vi "runtime test.vi"() -> (0 "error out":errorcluster, 2 "success?":bool)   [LabVIEW 2014, in "Shared Memory tests.lvlib"]
uses:
  Shared Memory tests.lvlib
  module/execution/Shared Memory runtime.lvclass
  <vilib>/NI/Tag Bus Module Framework/channel/channel classification.ctl
  module/execution/Shared Memory runtime.lvclass/Shared Memory runtime.ctl
  <vilib>/NI/NI Linux RT IPC/Shared Memory/Pointer Operations/Read 1D Array DBL.vi
  <vilib>/NI/Tag Bus/table/write multiple elements.vi
  <vilib>/NI/Tag Bus/table/data polymorphs/write many/write Doubles.vi
  <vilib>/NI/NI Linux RT IPC/Shared Memory/Pointer Operations/Read 1D Array SGL.vi
  <vilib>/NI/Tag Bus/table/data polymorphs/write many/write Singles.vi
  <vilib>/NI/NI Linux RT IPC/Shared Memory/Pointer Operations/Read 1D Array I64.vi
  <vilib>/NI/Tag Bus/table/data polymorphs/write many/write I64s.vi
  <vilib>/NI/NI Linux RT IPC/Shared Memory/Pointer Operations/Read 1D Array I32.vi
  <vilib>/NI/Tag Bus/table/data polymorphs/write many/write I32s.vi
  <vilib>/NI/NI Linux RT IPC/Shared Memory/Pointer Operations/Read 1D Array I16.vi
  <vilib>/NI/Tag Bus/table/data polymorphs/write many/write I16s.vi
  <vilib>/NI/NI Linux RT IPC/Shared Memory/Pointer Operations/Read 1D Array I8.vi
  <vilib>/NI/Tag Bus/table/data polymorphs/write many/write I8s.vi
  <vilib>/NI/NI Linux RT IPC/Shared Memory/Pointer Operations/Read 1D Array U64.vi
  <vilib>/NI/Tag Bus/table/data polymorphs/write many/write U64s.vi
  <vilib>/NI/NI Linux RT IPC/Shared Memory/Pointer Operations/Read 1D Array U32.vi
  <vilib>/NI/Tag Bus/table/data polymorphs/write many/write U32s.vi
  <vilib>/NI/NI Linux RT IPC/Shared Memory/Pointer Operations/Read 1D Array U16.vi
  <vilib>/NI/Tag Bus/table/data polymorphs/write many/write U16s.vi
  <vilib>/NI/NI Linux RT IPC/Shared Memory/Pointer Operations/Read 1D Array U8.vi
  <vilib>/NI/Tag Bus/table/data polymorphs/write many/write U8s.vi
  <vilib>/NI/NI Linux RT IPC/Shared Memory/Pointer Operations/Read 1D Array Boolean.vi
  <vilib>/NI/Tag Bus/table/data polymorphs/write many/write Booleans.vi
  <vilib>/NI/Tag Bus/table/write sequential data elements.vi
  <vilib>/NI/Tag Bus/table/data polymorphs/write sequential/write sequential Doubles.vi
  <vilib>/NI/Tag Bus/table/data polymorphs/write sequential/write sequential Singles.vi
  <vilib>/NI/Tag Bus/table/data polymorphs/write sequential/write sequential I64s.vi
  <vilib>/NI/Tag Bus/table/data polymorphs/write sequential/write sequential I32s.vi
  <vilib>/NI/Tag Bus/table/data polymorphs/write sequential/write sequential I16s.vi
  <vilib>/NI/Tag Bus/table/data polymorphs/write sequential/write sequential I8s.vi
  <vilib>/NI/Tag Bus/table/data polymorphs/write sequential/write sequential U64s.vi
  <vilib>/NI/Tag Bus/table/data polymorphs/write sequential/write sequential U32s.vi
  <vilib>/NI/Tag Bus/table/data polymorphs/write sequential/write sequential U16s.vi
  <vilib>/NI/Tag Bus/table/data polymorphs/write sequential/write sequential U8s.vi
  <vilib>/NI/Tag Bus/table/data polymorphs/write sequential/write sequential Booleans.vi
  module/execution/read channels of classification.vi
  <vilib>/NI/Tag Bus/table/read multiple elements.vi
  <vilib>/NI/Tag Bus/table/data polymorphs/read many/read Doubles.vi
  <vilib>/NI/NI Linux RT IPC/Shared Memory/Pointer Operations/Write 1D Array DBL.vi
  <vilib>/NI/Tag Bus/table/data polymorphs/read many/read Singles.vi
  <vilib>/NI/NI Linux RT IPC/Shared Memory/Pointer Operations/Write 1D Array SGL.vi
  <vilib>/NI/Tag Bus/table/data polymorphs/read many/read I64s.vi
  <vilib>/NI/NI Linux RT IPC/Shared Memory/Pointer Operations/Write 1D Array I64.vi
  <vilib>/NI/Tag Bus/table/data polymorphs/read many/read I32s.vi
  <vilib>/NI/NI Linux RT IPC/Shared Memory/Pointer Operations/Write 1D Array I32.vi
  <vilib>/NI/Tag Bus/table/data polymorphs/read many/read I16s.vi
  <vilib>/NI/NI Linux RT IPC/Shared Memory/Pointer Operations/Write 1D Array I16.vi
  <vilib>/NI/Tag Bus/table/data polymorphs/read many/read I8s.vi
  <vilib>/NI/NI Linux RT IPC/Shared Memory/Pointer Operations/Write 1D Array I8.vi
  <vilib>/NI/Tag Bus/table/data polymorphs/read many/read U64s.vi
  <vilib>/NI/NI Linux RT IPC/Shared Memory/Pointer Operations/Write 1D Array U64.vi
  <vilib>/NI/Tag Bus/table/data polymorphs/read many/read U32s.vi
  <vilib>/NI/NI Linux RT IPC/Shared Memory/Pointer Operations/Write 1D Array U32.vi
  <vilib>/NI/Tag Bus/table/data polymorphs/read many/read U16s.vi
  <vilib>/NI/NI Linux RT IPC/Shared Memory/Pointer Operations/Write 1D Array U16.vi
  <vilib>/NI/Tag Bus/table/data polymorphs/read many/read U8s.vi
  <vilib>/NI/NI Linux RT IPC/Shared Memory/Pointer Operations/Write 1D Array U8.vi
  <vilib>/NI/Tag Bus/table/data polymorphs/read many/read Booleans.vi
  <vilib>/NI/NI Linux RT IPC/Shared Memory/Pointer Operations/Write 1D Array Boolean.vi
  <vilib>/NI/Tag Bus/table/read sequential data elements.vi
  <vilib>/NI/Tag Bus/table/data polymorphs/read sequential/read sequential Doubles.vi
  <vilib>/NI/Tag Bus/table/data polymorphs/read sequential/read sequential Singles.vi
  <vilib>/NI/Tag Bus/table/data polymorphs/read sequential/read sequential I64s.vi
  <vilib>/NI/Tag Bus/table/data polymorphs/read sequential/read sequential I32s.vi
  <vilib>/NI/Tag Bus/table/data polymorphs/read sequential/read sequential I16s.vi
  <vilib>/NI/Tag Bus/table/data polymorphs/read sequential/read sequential I8s.vi
  <vilib>/NI/Tag Bus/table/data polymorphs/read sequential/read sequential U64s.vi
  <vilib>/NI/Tag Bus/table/data polymorphs/read sequential/read sequential U32s.vi
  <vilib>/NI/Tag Bus/table/data polymorphs/read sequential/read sequential U16s.vi
  <vilib>/NI/Tag Bus/table/data polymorphs/read sequential/read sequential U8s.vi
  <vilib>/NI/Tag Bus/table/data polymorphs/read sequential/read sequential Booleans.vi
  module/execution/Read input data.vi
  module/execution/Read processing parameters.vi
  module/execution/Read processing results.vi
  module/execution/Read output data.vi
  <vilib>/NI/NI Linux RT IPC/Shared Memory/Classes/Shared Memory/Shared Memory.lvclass
  module/configuration/Shared Memory configuration.lvclass
  <vilib>/NI/Tag Bus Module Framework/channel/TBM channel.lvclass
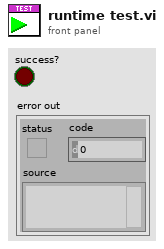
[diagram p1: front panel]
types:
  T1 = typedef "TBM channel.lvclass/channel classification.ctl" = enum16{"input data", "output data", "processing parameter", "processing result"}
  T2 = typedef "TBM channel.lvclass/data tables.ctl" = cluster{"input data":T3, "processing parameter":T3, "processing result":T3, "output data":T3}
  T3 = typedef "tag bus.lvlib/dictionary table pair.ctl" = cluster{"data dictionary":refnum<class "data dictionary.lvclass">, "data table":T4}
  T4 = typedef "tag bus.lvlib/data table.lvlib/data table.ctl" = cluster{"Double":dbl[], "Single":sgl[], "I64":i64[], "I32":i32[], "I16":i16[], "I8":i8[], "U64":u64[], "U32":u32[], "U16":u16[], "U8":u8[], "Boolean":bool[], "String":string[], "Array of Double":cluster{"DBL Array":dbl[]}[], "Array of Single":cluster{"SGL Array":sgl[]}[], "Array of I64":cluster{"I64 Array":i64[]}[], "Array of I32":cluster{"I32 Array":i32[]}[], "Array of I16":cluster{"I16 Array":i16[]}[], "Array of I8":cluster{"I8 Array":i8[]}[], "Array of U64":cluster{"U64 Array":u64[]}[], "Array of U32":cluster{"U32 Array":u32[]}[], "Array of U16":cluster{"U16 Array":u16[]}[], "Array of U8":cluster{"U8 Array":u8[]}[], "Array of Boolean":cluster{"Boolean Array":bool[]}[], "Array of String":cluster{"String Array":string[]}[]}
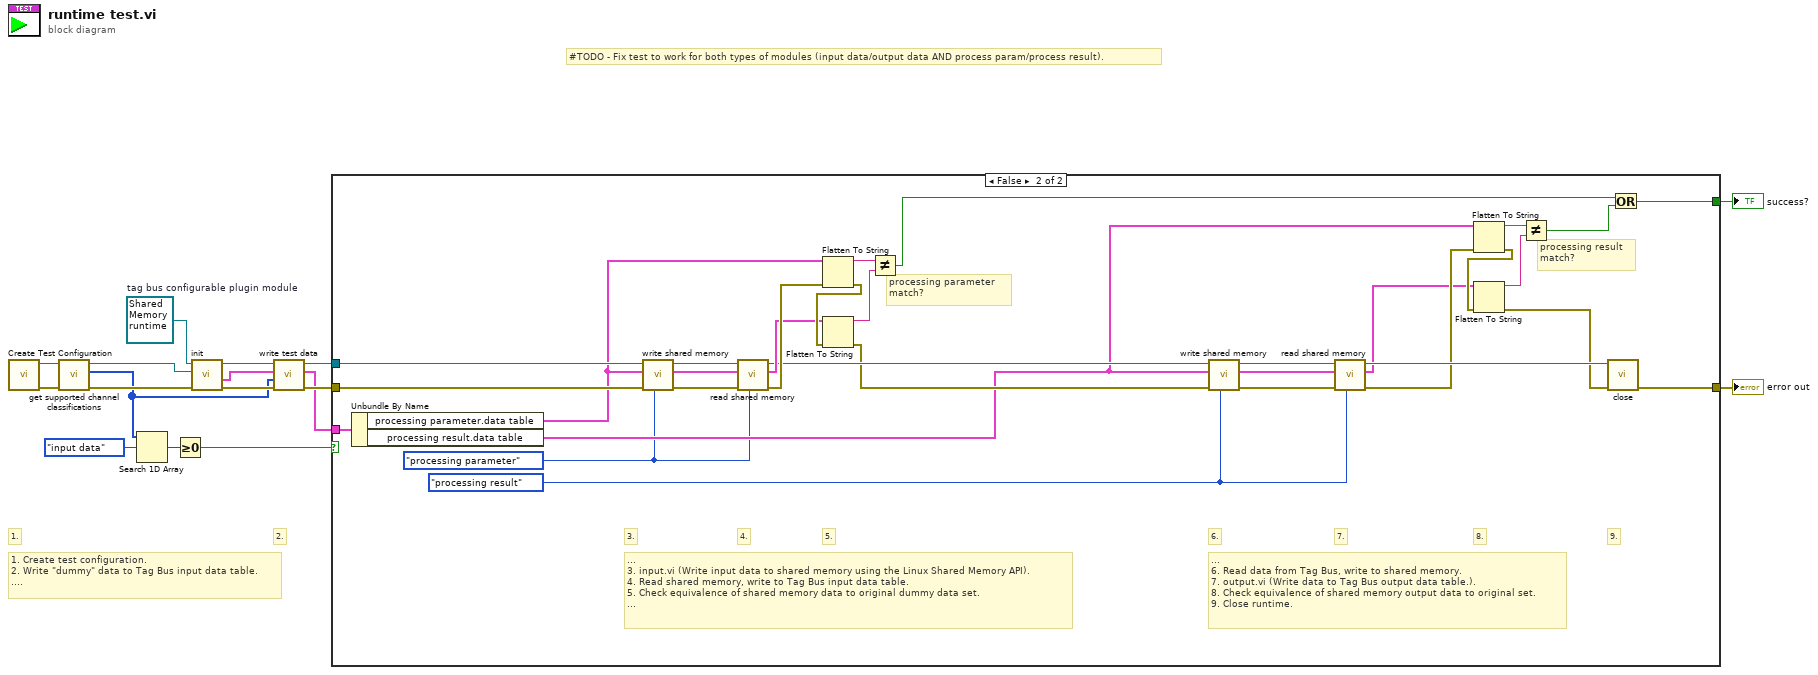
[diagram p0: block diagram]
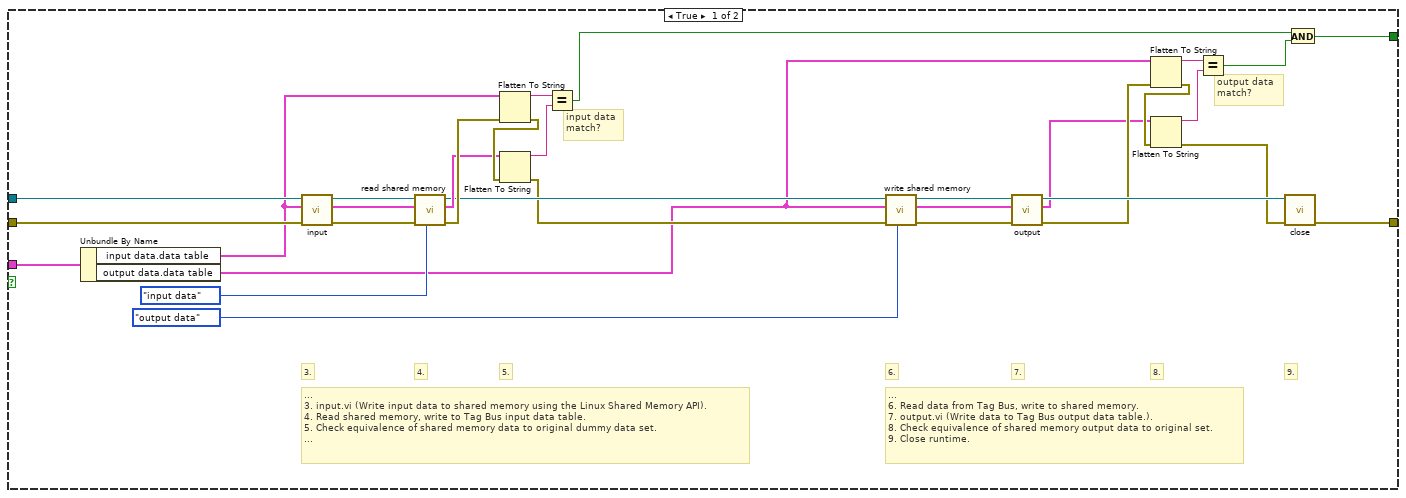
[diagram p2: hidden frame]
diagram:
  w13 = refnum<class "Shared Memory runtime.lvclass"> refnum  # tag bus configurable plugin module
  # "#TODO - Fix test to work for both types of modules (input data/output data AND process param/process result)."
  # "2."
  # "1. Create test configuration.\n2. Write \"dummy\" data to Tag Bus input data table.\n...."
  # "1."
  n1 = call "Create Test Configuration.vi"() -> ("error out"=w15:errorcluster, "Module Configuration"=w14:refnum<class "Shared Memory configuration.lvclass">)  [unwired: 3 in, 7 out]
  n2 = call-dynamic "get supported channel classifications.vi"("error in"=w15, "module configuration in"=w14) -> ("error out"=w12:errorcluster, "supported classes"=w5:T1[], "module configuration out"=w11:refnum<class "Shared Memory configuration.lvclass">)  [unwired: 7 in]
  n3 = Search 1D Array(1D array=w5, element=channel_classification."input data" ("channel classification")) -> (index of element=w3:i32)  [unwired: 1 in]
  n4 = Greater Or Equal To 0?(x=w3) -> (x >= 0?=w1:bool)
  n5 = call-dynamic "init.vi"("error in"=w12, "TBM module configuration in"=w11, "Shared Memory runtime in"=w13) -> ("error out"=w8:errorcluster, "data allocations"=w6:T2, "Shared Memory runtime out"=w7:refnum<class "Shared Memory runtime.lvclass">)  [unwired: 5 in, 1 out]
  n6 = call "write test data.vi"("shared memory runtime"=w7, "data allocations"=w6, "supported classifications"=w5, "error in"=w8) -> ("shared memory runtime out"=w9:refnum<class "Shared Memory runtime.lvclass">, "data allocations out"=w2:T2, "error out"=w10:errorcluster)  [unwired: 4 in]
  n7 = case shown="False" w1 {
    tunnel: [w48 w79] -> w17
    tunnel: [w47 w78] -> w16
    tunnel: w10 -> [w42 w54]
    tunnel: w9 -> [w41 w56]
    tunnel: w2 -> [w19 w58]
    frame True {
      # "output data\nmatch?"
      # "input data\nmatch?"
      # "...\n6. Read data from Tag Bus, write to shared memory.\n7. output.vi (Write data to Tag Bus output data table.).\n8. Check equivalence of shared memory output data to original set.\n9. Close runtime."
      # "...\n3. input.vi (Write input data to shared memory using the Linux Shared Memory API).\n4. Read shared memory, write to Tag Bus input data table.\n5. Check equivalence of shared memory data to original dummy data set.\n..."
      # "6."
      # "5."
      # "7."
      # "4."
      # "3."
      # "8."
      # "9."
      n8 = Unbundle By Name(w19) -> ("input data.data table"=w20:T4, "output data.data table"=w18:T4)
      n9 = call-dynamic "input.vi"("error in"=w42, "data table in"=w20, "Shared Memory runtime in"=w41) -> ("error out"=w37:errorcluster, "data table out"=w31:T4, "Shared Memory runtime out"=w36:refnum<class "Shared Memory runtime.lvclass">)  [unwired: 6 in]
      n10 = call "read shared memory.vi"("channel classification"=channel_classification."input data", "error in"=w37, "data table"=w31, "Shared Memory runtime"=w36) -> ("error out"=w35:errorcluster, "data table out"=w34:T4, "Shared Memory runtime out"=w33:refnum<class "Shared Memory runtime.lvclass">)  [unwired: 5 in]
      n11 = Flatten To String(anything=w20, error in (no error)=w35) -> (data string=w40:string, error out=w38:errorcluster)  [unwired: 2 in, 1 out]
      n12 = Flatten To String(anything=w34, error in (no error)=w38) -> (data string=w39:string, error out=w32:errorcluster)  [unwired: 2 in, 1 out]
      n13 = Equal?(x=w40, y=w39) -> (x = y?=w45:bool)
      n14 = call "write shared memory.vi"("channel classification"=channel_classification."output data", "error in"=w32, "data table"=w18, "module in"=w33) -> ("error out"=w29:errorcluster, "data table out"=w23:T4, "module out"=w30:refnum<class "Shared Memory runtime.lvclass">)  [unwired: 5 in]
      n15 = call-dynamic "output.vi"("error in"=w29, "data table in"=w23, "Shared Memory runtime in"=w30) -> ("error out"=w25:errorcluster, "data table out"=w24:T4, "Shared Memory runtime out"=w46:refnum<class "Shared Memory runtime.lvclass">)  [unwired: 6 in]
      n16 = Flatten To String(anything=w18, error in (no error)=w25) -> (data string=w26:string, error out=w28:errorcluster)  [unwired: 2 in, 1 out]
      n17 = Flatten To String(anything=w24, error in (no error)=w28) -> (data string=w27:string, error out=w43:errorcluster)  [unwired: 2 in, 1 out]
      n18 = Equal?(x=w26, y=w27) -> (x = y?=w44:bool)
      n19 = call-dynamic "close.vi"("error in"=w43, "Shared Memory runtime in"=w46) -> ("error out"=w48:errorcluster)  [unwired: 9 in]
      n20 = And(x=w45, y=w44) -> (x .and. y?=w47:bool)
    }
    frame False {
      w50 = channel_classification."processing result" ("channel classification")
      w52 = channel_classification."processing parameter" ("channel classification")
      # "processing result\nmatch?"
      # "processing parameter\nmatch?"
      # "...\n6. Read data from Tag Bus, write to shared memory.\n7. output.vi (Write data to Tag Bus output data table.).\n8. Check equivalence of shared memory output data to original set.\n9. Close runtime."
      # "...\n3. input.vi (Write input data to shared memory using the Linux Shared Memory API).\n4. Read shared memory, write to Tag Bus input data table.\n5. Check equivalence of shared memory data to original dummy data set.\n..."
      # "6."
      # "5."
      # "7."
      # "4."
      # "3."
      # "8."
      # "9."
      n21 = Unbundle By Name(w58) -> ("processing parameter.data table"=w49:T4, "processing result.data table"=w57:T4)
      n22 = call "write shared memory.vi"("channel classification"=w52, "error in"=w54, "data table"=w49, "module in"=w56) -> ("error out"=w53:errorcluster, "data table out"=w51:T4, "module out"=w55:refnum<class "Shared Memory runtime.lvclass">)  [unwired: 5 in]
      n23 = call "read shared memory.vi"("channel classification"=w52, "error in"=w53, "data table"=w51, "Shared Memory runtime"=w55) -> ("error out"=w70:errorcluster, "data table out"=w69:T4, "Shared Memory runtime out"=w68:refnum<class "Shared Memory runtime.lvclass">)  [unwired: 5 in]
      n24 = Flatten To String(anything=w49, error in (no error)=w70) -> (data string=w73:string, error out=w71:errorcluster)  [unwired: 2 in, 1 out]
      n25 = Flatten To String(anything=w69, error in (no error)=w71) -> (data string=w72:string, error out=w67:errorcluster)  [unwired: 2 in, 1 out]
      n26 = Not Equal?(x=w73, y=w72) -> (x != y?=w76:bool)
      n27 = call "write shared memory.vi"("channel classification"=w50, "error in"=w67, "data table"=w57, "module in"=w68) -> ("error out"=w65:errorcluster, "data table out"=w59:T4, "module out"=w66:refnum<class "Shared Memory runtime.lvclass">)  [unwired: 5 in]
      n28 = call "read shared memory.vi"("channel classification"=w50, "error in"=w65, "data table"=w59, "Shared Memory runtime"=w66) -> ("error out"=w61:errorcluster, "data table out"=w60:T4, "Shared Memory runtime out"=w77:refnum<class "Shared Memory runtime.lvclass">)  [unwired: 5 in]
      n29 = Flatten To String(anything=w57, error in (no error)=w61) -> (data string=w62:string, error out=w64:errorcluster)  [unwired: 2 in, 1 out]
      n30 = Flatten To String(anything=w60, error in (no error)=w64) -> (data string=w63:string, error out=w74:errorcluster)  [unwired: 2 in, 1 out]
      n31 = Not Equal?(x=w62, y=w63) -> (x != y?=w75:bool)
      n32 = call-dynamic "close.vi"("error in"=w74, "Shared Memory runtime in"=w77) -> ("error out"=w79:errorcluster)  [unwired: 9 in]
      n33 = Or(x=w76, y=w75) -> (x .or. y?=w78:bool)
    }
  }
  "error out" <- w17
  "success?" <- w16
